vi "Read System Errors.vi"(8 "error in (no error)":errorcluster, 11 "PAS Data in":refnum<class "PAS Data.lvclass">) -> (0 "error out":errorcluster, 2 "System Errors":T1, 3 "PAS Data out":refnum<class "PAS Data.lvclass">)   [LabVIEW 2014, in "PAS Data.lvclass"]
doc: "Retrieve errors from the PAS that may result in unexpected behavior of instrument or in incorrect retrieval of data."
uses:
  PAS Data.lvclass
  PAS Data.lvclass/PAS Data.ctl
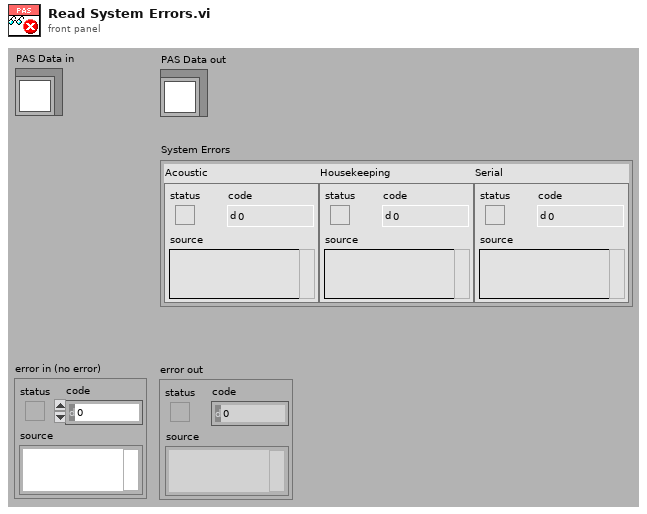
[diagram p1: front panel]
types:
  T1 = cluster{"Acoustic ":errorcluster, "Housekeeping":errorcluster, "Serial":errorcluster}
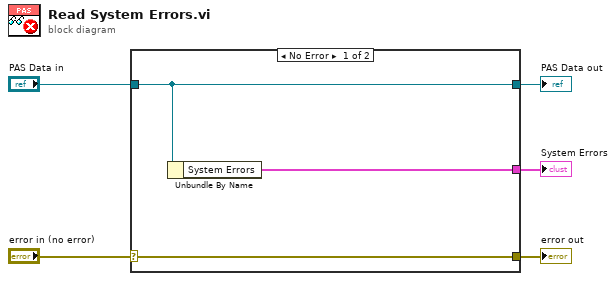
[diagram p0: block diagram]
diagram:
  n1 = case shown="No Error" "error in (no error)" {
    selector: "error in (no error)" -> [w8 w9]
    tunnel: [w8 w9] -> w4
    tunnel: [w7 w10] -> w2
    tunnel: "PAS Data in" -> [w7 w10]
    tunnel: [w6 _] -> w1
    frame No Error {
      n2 = Unbundle By Name(w7) -> ("System Errors"=w6:T1)
    }
    frame Error {
    }
  }
  "error out" <- w4
  "PAS Data out" <- w2
  "System Errors" <- w1
